vi "Init Events.vi"(8 "error in (no error)":errorcluster, 11 "Log_Engine in":refnum<class "Log_Engine.lvclass">) -> (0 "error out":errorcluster, 3 "Log_Engine out":refnum<class "Log_Engine.lvclass">)   [LabVIEW 2019, in "Log_Engine.lvclass"]
doc: "Developed by Kevin Thompson\nkevin@thompsonengineering.net\n\nCopyright 2018\nThompson Engineering, LLC"
uses:
  Log_Engine.lvclass
  Common/DataTypes/TD Async CmdMsg EventData--cluster.ctl
  DataTypes/LogStateChg EvData--cluster.ctl
  DataTypes/LogStateEvData--cluster.ctl
  Common/DataTypes/LogState--enum.ctl
  DataTypes/TDMSStateChg EvData--cluster.ctl
  DataTypes/TDMSStateEvData--cluster.ctl
  Common/DataTypes/TDMSState--enum.ctl
  Log_Engine.lvclass/Log_Engine.ctl
  Accessors/Get PublicEvents.vi
  Accessors/Set PublicEvents.vi
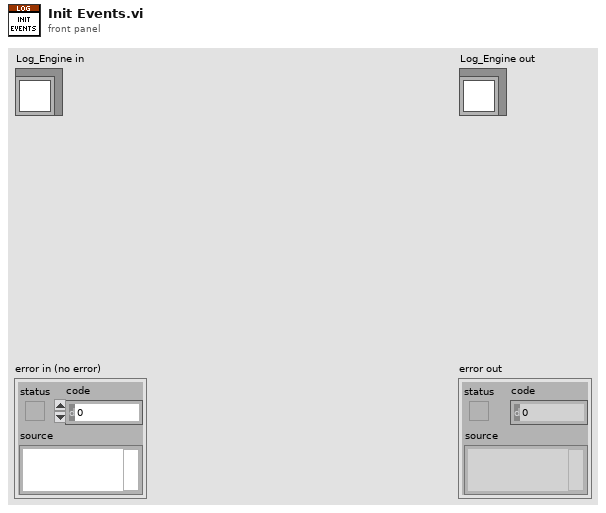
[diagram p1: front panel]
types:
  T1 = typedef "Log_Engine.lvclass/TDMSStateChg EvData--cluster.ctl" = cluster{"Time Stamp":timestamp, "OLD State":T2, "NEW State":T2}
  T2 = typedef "Log_Engine.lvclass/TDMSStateEvData--cluster.ctl" = cluster{"TDMSState":T3, "vData":variant}
  T3 = typedef "TDMSState--enum.ctl" = enum16{"Unknown", "Stopped", "Running", "Error"}
  T4 = typedef "Log_Engine.lvclass/LogStateChg EvData--cluster.ctl" = cluster{"Time Stamp":timestamp, "OLD State":T5, "NEW State":T5}
  T5 = typedef "Log_Engine.lvclass/LogStateEvData--cluster.ctl" = cluster{"LogState":T6, "vData":variant}
  T6 = typedef "LogState--enum.ctl" = enum16{"Unknown", "Stopped", "Running", "Error"}
  T7 = typedef "TD Async CmdMsg EventData--cluster.ctl" = cluster{"Time Stamp":timestamp, "CmdMsg":string, "vData":variant}
  T8 = typedef "Log_Engine.lvclass/Public Events--cluster.ctl" = cluster{"Log_Engine.AsyncCmd Event":refnum<user-event>, "Log_Engine.AsyncMsg Event":refnum<user-event>, "stop process":refnum<user-event>, "Log_Engine.LogStateChg Ev":refnum<user-event>, "Log_Engine.TDMSStateChg Ev":refnum<user-event>}
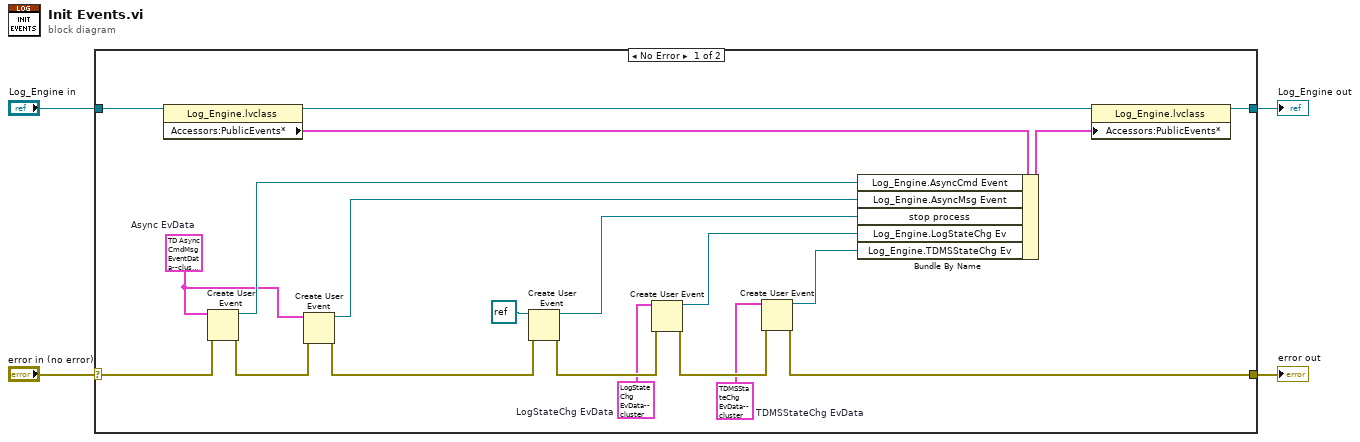
[diagram p0: block diagram]
diagram:
  n1 = case shown="No Error" "error in (no error)" {
    selector: "error in (no error)" -> [w16 w26]
    tunnel: [w10 w26] -> w3
    tunnel: [w24 w25] -> w1
    tunnel: "Log_Engine in" -> [w23 w25]
    frame No Error {
      w6 = T1 {"Time Stamp"=timestamp(0 s since 1904-01-01), "OLD State"={"TDMSState"=enum."Unknown", "vData"=variant}, "NEW State"={"TDMSState"=enum."Unknown", "vData"=variant}}  # TDMSStateChg EvData
      w8 = T4 {"Time Stamp"=timestamp(0 s since 1904-01-01), "OLD State"={"LogState"=enum."Unknown", "vData"=variant}, "NEW State"={"LogState"=enum."Unknown", "vData"=variant}}  # LogStateChg EvData
      w13 = T7 {"Time Stamp"=timestamp(0 s since 1904-01-01), "CmdMsg"="", "vData"=variant}  # Async EvData
      n2 = property class="Log_Engine.lvclass"(reference=w23) -> (reference out=w22:refnum<class "Log_Engine.lvclass">, "Accessors:PublicEvents*"=w21:T8)  [unwired: 1 in, 1 out]
      n3 = Create User Event(user event datatype=w13, error in=w16) -> (user event=w17:refnum<user-event>, error out=w15:errorcluster)
      n4 = Create User Event(user event datatype=w13, error in=w15) -> (user event=w12:refnum<user-event>, error out=w14:errorcluster)
      n5 = Create User Event(user event datatype=refnum<notifier> refnum ("notifier out"), error in=w14) -> (user event=w18:refnum<user-event>, error out=w11:errorcluster)
      n6 = Create User Event(user event datatype=w8, error in=w11) -> (user event=w7:refnum<user-event>, error out=w9:errorcluster)
      n7 = Create User Event(user event datatype=w6, error in=w9) -> (user event=w5:refnum<user-event>, error out=w10:errorcluster)
      n8 = Bundle By Name(cluster=w21, "Log_Engine.AsyncCmd Event"=w17, "Log_Engine.AsyncMsg Event"=w12, "stop process"=w18, "Log_Engine.LogStateChg Ev"=w7, "Log_Engine.TDMSStateChg Ev"=w5) -> (w20:T8)
      n9 = property class="Log_Engine.lvclass"(reference=w22, "Accessors:PublicEvents*"=w20) -> (reference out=w24:refnum<class "Log_Engine.lvclass">)  [unwired: 1 in, 1 out]
    }
    frame Error {
    }
  }
  "error out" <- w3
  "Log_Engine out" <- w1
